vi "ReadSecuence.vi"() -> (1 "ACQType":T1 items=["Digital", "Analog"], 2 "AnalogConfig":T2, 3 "DigitalConfig":T3)   [LabVIEW 2020, in "Settings.lvlib"]
uses:
  Settings.lvlib
  Acquisition/DigitalConfig--cluster.ctl
  Acquisition/AnalogConfig--cluster.ctl
  Downloads/ProyFinSAD_PabloCesarRamosE/EnumTypeDef.ctl
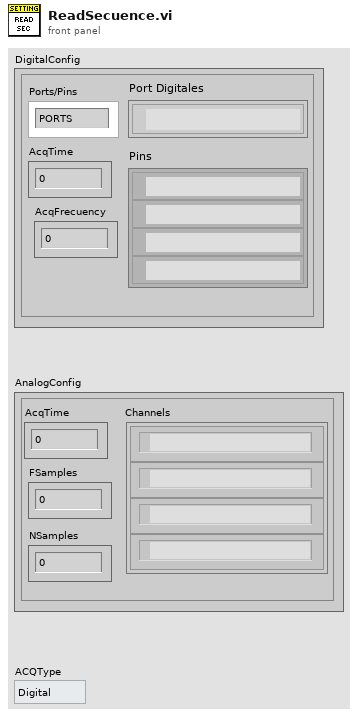
[diagram p1: front panel]
types:
  T1 = typedef "EnumTypeDef.ctl" = u16
  T2 = typedef "AnalogConfig--cluster.ctl" = cluster{"AcqTime":dbl, "FSamples":dbl, "NSamples":dbl, "Channels":tag[]}
  T3 = typedef "DigitalConfig--cluster.ctl" = cluster{"Ports/Pins":enum16{"PORTS", "PINS"}, "AcqTime":dbl, "AcqFrecuency":dbl, "Port Digitales":tag[], "Pins":tag[]}
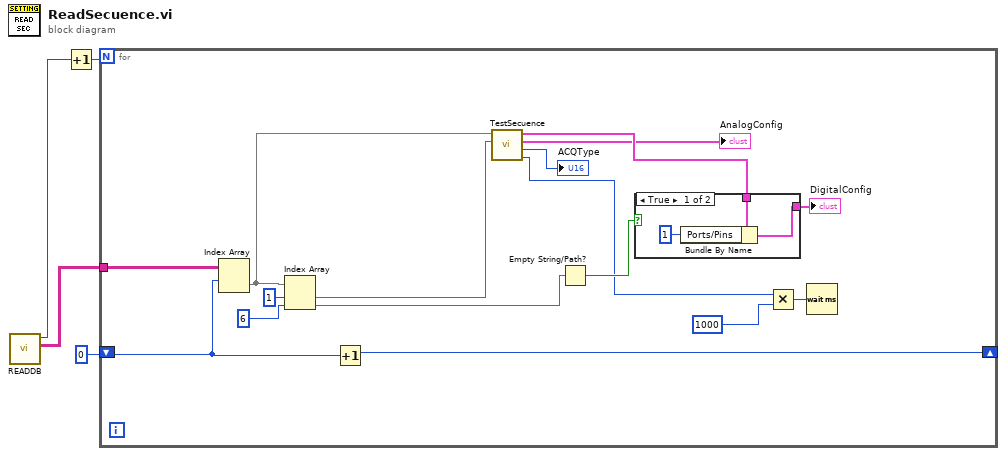
[diagram p0: block diagram]
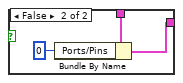
[diagram p2: hidden frame]
diagram:
  n1 = call "READDB.vi"() -> ("Datos"=w3:string[][], "Max ID"=w1:i32)  [unwired: 8 in, 2 out]
  n2 = Increment(x=w1) -> (x+1=w2:i32)
  n3 = for {
    N: w2 -> [_]
    shift-right: [w15] -> _
    shift-left: 0 -> [w14]
    tunnel: w3 -> [w13]
    n4 = Index Array(array=w13, index (row)=w14) -> (element=w12:string[])  [unwired: 1 in]
    n5 = Index Array(array=w12, index #1=1 ("index"), index #2=6 ("index")) -> (element #1=w11:string, element #2=w20:string)
    n6 = Increment(x=w14) -> (x+1=w15:i32)
    n7 = call "TestSecuence.vi"("String"=w11, "Result Set"=w12) -> ("Time"=w9:i32, "ACQType"=→"ACQType":T1, "AnalogConfig"=→"AnalogConfig":T2, "DigitalConfig"=w8:T3)  [unwired: 6 in]
    n8 = Empty String/Path?(string/path=w20) -> (empty?=w10:bool)
    n9 = case shown="True" w10 {
      tunnel: w8 -> [w23 w26]
      tunnel: [w22 w25] -> w7
      frame True {
        n10 = Bundle By Name(cluster=w23, "Ports/Pins"=u16 1) -> (w22:T3)
      }
      frame False {
        n11 = Bundle By Name(cluster=w26, "Ports/Pins"=u16 0) -> (w25:T3)
      }
    }
    "DigitalConfig" <- w7
    n12 = Multiply(x=w9, y=1000) -> (x*y=w16:i32)
    n13 = Wait (ms)(milliseconds to wait=w16) -> ()  [unwired: 1 out]
  }
